vi "pub_multipart.vi"() -> ()   [LabVIEW 2014]
uses:
  lvnanomsg/socket_type.ctl
  lvnanomsg/nanomsg_context.lvclass
  lvnanomsg/nanomsg_socket.lvclass
  lvnanomsg/nanomsg.lvlib
panel:
  out "message":string[](array[string])
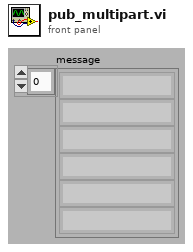
[diagram p1: front panel]
types:
  T1 = typedef "nanomsg.lvlib/socket_type.ctl" = enum8{"NN_SOL_SOCKET", "NN_1", "NN_2", "NN_3", "NN_4", "NN_5", "NN_6", "NN_7", "NN_8", "NN_9", "NN_10", "NN_11", "NN_12", "NN_13", "NN_14", "NN_15", "NN_PAIR", "NN_17", "NN_18", "NN_19", "NN_20", "NN_21", "NN_22", "NN_23", "NN_24", "NN_25", "NN_26", "NN_27", "NN_28", "NN_29", "NN_30", "NN_31", "NN_PUB", "NN_SUB", "NN_34", "NN_35", "NN_36", "NN_37", "NN_38", "NN_39", "NN_40", "NN_41", "NN_42", "NN_43", "NN_44", "NN_45", "NN_46", "NN_47", "REQ_REQ", "REP_REP", "NN_50", "NN_51", "NN_52", "NN_53", "NN_54", "NN_55", "NN_56", "NN_57", "NN_58", "NN_59", "NN_60", "NN_61", "NN_62", "NN_63", "NN_64", "NN_65", "NN_66", "NN_67", "NN_68", "NN_69", "NN_70", "NN_71", "NN_72", "NN_73", "NN_74", "NN_75", "NN_76", "NN_77", "NN_78", "NN_79", "NN_PUSH", "NN_PULL", "NN_82", "NN_83", "NN_84", "NN_85", "NN_86", "NN_87", "NN_88", "NN_89", "NN_90", "NN_91", "NN_92", "NN_93", "NN_94", "NN_95", "NN_96", "NN_97", "NN_SURVEYOR", "NN_RESPONDENT", "NN_100", "NN_101", "NN_102", "NN_103", "NN_104", "NN_105", "NN_106", "NN_107", "NN_108", "NN_109", "NN_110", "NN_111", "NN_BUS"}
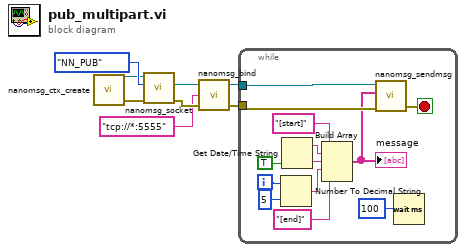
[diagram p0: block diagram]
diagram:
  n1 = call "nanomsg_ctx_create.vi"() -> ("error out"=w6:errorcluster, "context out"=w3:refnum<class "nanomsg_context.lvclass">)  [unwired: 4 in]
  n2 = call "nanomsg_socket.vi"("error in"=w6, "socket type"=socket_type."NN_PUB", "context in"=w3) -> ("error out"=w5:errorcluster, "socket out"=w2:refnum<class "nanomsg_socket.lvclass">)  [unwired: 2 in, 1 out]
  n3 = call "nanomsg_bind.vi"("error in"=w5, "endpoint"="tcp://*:5555", "socket in"=w2) -> ("error out"=w4:errorcluster, "socket out"=w8:refnum<class "nanomsg_socket.lvclass">)  [unwired: 1 in]
  n4 = while {
    tunnel: w8 -> [w20]
    tunnel: w4 -> [w19]
    i -> [w10]
    stop <- w18 stop-if-true
    n5 = Number To Decimal String(number=w10, width (-)=5) -> (decimal integer string=w12:string)
    n6 = Get Date/Time String(want seconds? (F)=TRUE) -> (date string=w17:string, time string=w16:string)  [unwired: 2 in]
    n7 = Build Array("[start]" ("element"), w17, w16, w12, "[end]" ("element")) -> (w14:string[])
    "message" <- w14
    n8 = call "nanomsg_sendmsg.vi"("error in"=w19, "parts"=w14, "socket in"=w20) -> ("error out"=w18:errorcluster)  [unwired: 2 in, 1 out]
    n9 = Wait (ms)(milliseconds to wait=u32 100) -> ()  [unwired: 1 out]
  }
